vi "Stop Sift Proxy If Running.vi"(0 "Sift Client in":refnum<class "Sift Client.lvclass">, 5 "Address":string, 7 "Timeout":i32=1000, 11 "error in (no error)":errorcluster) -> (4 "Sift Client out":refnum<class "Sift Client.lvclass">, 6 "Success":bool, 15 "error out":errorcluster)   [LabVIEW 2024, in "Sift Client.lvlib" / "Sift Client.lvclass"]
uses:
  Sift Client.lvclass
  Generate Sift Protos/SiftProxy_client/RPC Messages/sift_proxy_v1_Empty_Flat.ctl
  0a8a573c-cadc-4f02-b59d-b76f69b4f265.vi
  Generate Sift Protos/SiftProxy_client/SiftProxy_client.lvlib
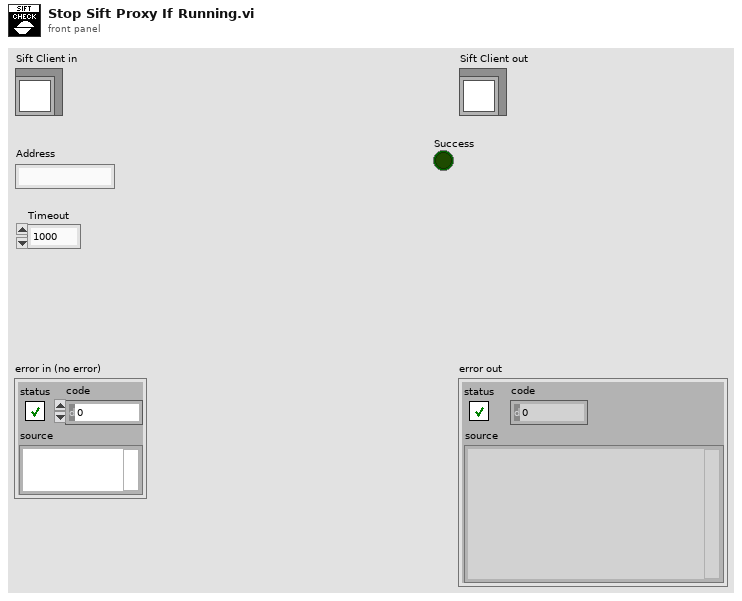
[diagram p1: front panel]
types:
  T1 = typedef "SiftProxy_client.lvlib/sift_proxy_v1_Empty_Flat.ctl" = cluster{"void":string}
  T2 = typedef "grpc-lvsupport-release.lvlib/grpcId.ctl" = u64
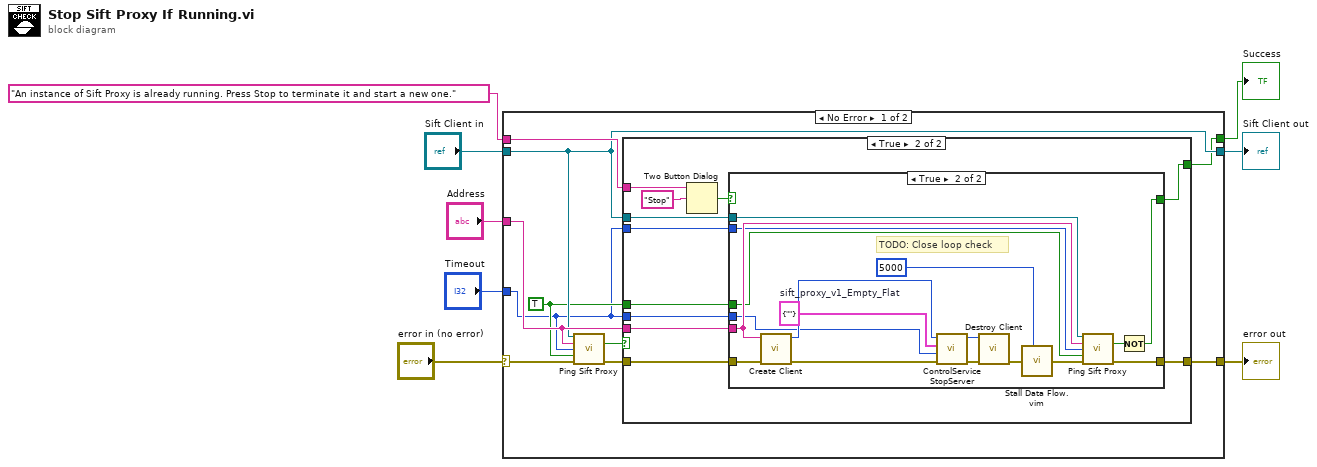
[diagram p0: block diagram]
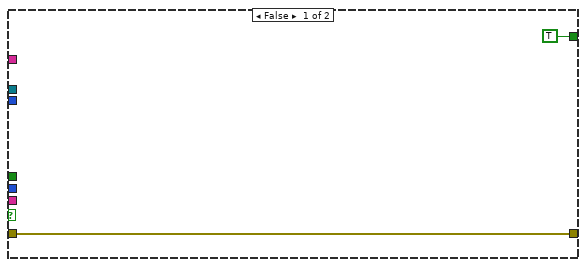
[diagram p2: hidden frame]
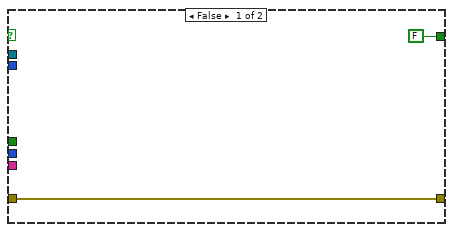
[diagram p3: hidden frame]
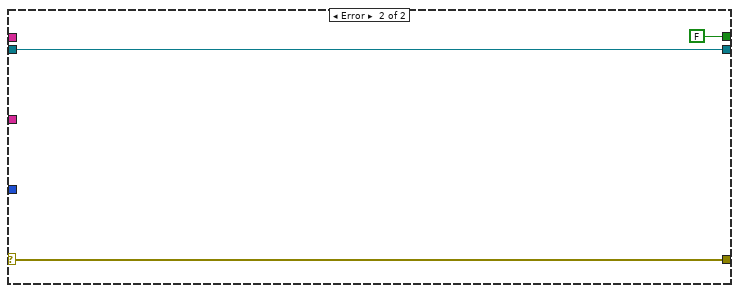
[diagram p4: hidden frame]
diagram:
  n1 = case shown="No Error" "error in (no error)" {
    selector: "error in (no error)" -> [w18 w53]
    tunnel: [w14 w53] -> w7
    tunnel: [w12 w52] -> w5
    tunnel: "Sift Client in" -> [w12 w52]
    tunnel: "Address" -> [w16 _]
    tunnel: [w10 FALSE] -> w3
    tunnel: "Timeout" -> [w9 _]
    tunnel: "An instance of Sift Proxy is already running. Press Stop to terminate it and start a new one." -> [w13 _]
    frame No Error {
      w11 = TRUE
      n2 = call-dynamic "Ping Sift Proxy.vi"("Sift Client in"=w12, "Address"=w16, "Timeout"=w9, "Destroy Client"=w11, "error in (no error)"=w18) -> ("Success"=w17:bool, "error out"=w15:errorcluster)  [unwired: 7 in, 2 out]
      n3 = case shown="True" w17 {
        tunnel: w16 -> [_ w31]
        tunnel: w15 -> [w19 w30]
        tunnel: [w19 w29] -> w14
        tunnel: w13 -> [_ w26]
        tunnel: w12 -> [_ w25]
        tunnel: w9 -> [_ w24]
        tunnel: w11 -> [_ w23]
        tunnel: [TRUE w22] -> w10
        tunnel: w9 -> [_ w21]
        frame False {
        }
        frame True {
          n4 = Two Button Dialog(message=w26, 2:"Stop") -> (T button?=w27:bool)  [unwired: 1 in]
          n5 = case shown="True" w27 {
            tunnel: w31 -> [_ w41]
            tunnel: w30 -> [w32 w46]
            tunnel: [w32 w37] -> w29
            tunnel: w25 -> [_ w42]
            tunnel: w24 -> [_ w40]
            tunnel: w23 -> [_ w39]
            tunnel: [FALSE w35] -> w22
            tunnel: w21 -> [_ w34]
            frame False {
            }
            frame True {
              w48 = T1 {"void"=""}  # sift_proxy_v1_Empty_Flat
              # "TODO: Close loop check"
              n6 = call "Create Client.vi"("error in"=w46, "address"=w41) -> ("error out"=w45:errorcluster, "gRPC ID Out"=w47:T2)  [unwired: 8 in]
              n7 = call "ControlService StopServer.vi"("error in"=w45, "timeout (ms)"=w34, "Request Data"=w48, "gRPC ID"=w47) -> ("error out"=w49:errorcluster, "gRPC ID out"=w50:T2)  [unwired: 5 in, 1 out]
              n8 = call "Destroy Client.vi"("error in"=w49, "gRPC ID"=w50) -> ("error out"=w44:errorcluster)  [unwired: 9 in]
              n9 = call "Stall Data Flow.vim"("value in"=w44, "milliseconds to wait"=5000) -> ("value out"=w38:errorcluster)  [unwired: 1 out]
              n10 = call-dynamic "Ping Sift Proxy.vi"("Sift Client in"=w42, "Address"=w41, "Timeout"=w40, "Destroy Client"=w39, "error in (no error)"=w38) -> ("Success"=w36:bool, "error out"=w37:errorcluster)  [unwired: 7 in, 2 out]
              n11 = Not(x=w36) -> (.not. x?=w35:bool)
            }
          }
        }
      }
    }
    frame Error {
    }
  }
  "error out" <- w7
  "Sift Client out" <- w5
  "Success" <- w3
